vi "Single Axis Controller.vi"(0 "Measured Value":sgl, 1 "Setpoint\nSource":T3(radio), 2 "Signal\nParameters":T2, 3 "Manual\nSetpoint":sgl(slide) scale=-10.0..10.0, 4 "Enable":T1, 5 "Gains":cluster{"P":sgl, "I":sgl, "D":sgl}={"P"=0.1, "I"=0.1, "D"=0.1}, 9 "Integral In":sgl) -> (11 "Integral Out":sgl, 14 "Controller \nOutput":sgl, 15 "Sepoint \nChart":cluster{sgl, "Setpoint out":sgl}(graph), 16 "Output\nComponents\nChart":cluster{sgl, sgl, sgl, sgl, sgl, sgl}(graph), 19 "Waveform Chart":cluster{sgl, sgl}(graph))   [LabVIEW 2014]
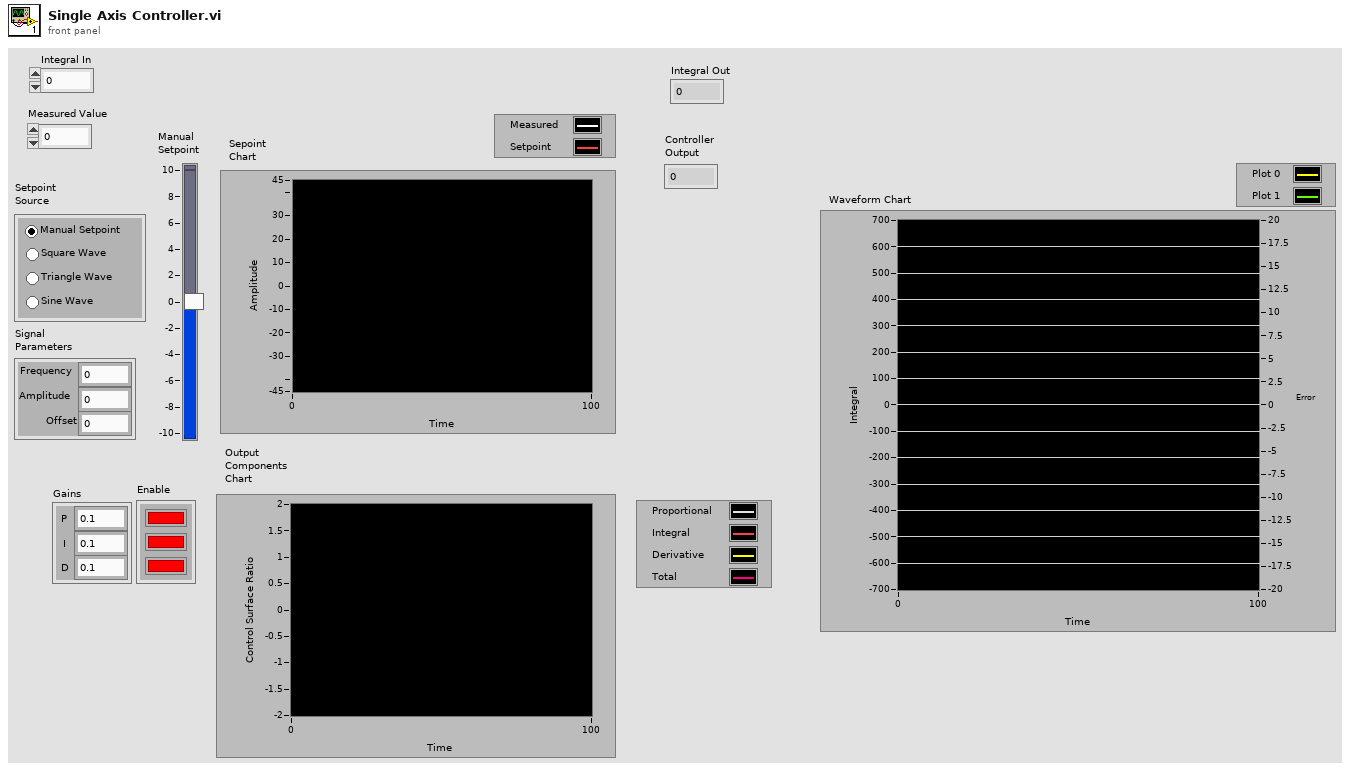
[diagram p1: front panel]
types:
  T1 = cluster{"P Enable":bool, "I Enable":bool, "D Enable":bool}
  T2 = cluster{"Frequency":sgl, "Amplitude":sgl, "Offset":sgl}
  T3 = enum32{"Manual Setpoint", "Square Wave", "Triangle Wave", "Sine Wave"}
  T4 = cluster{"Measured Value":sgl, "Setpoint out":sgl}
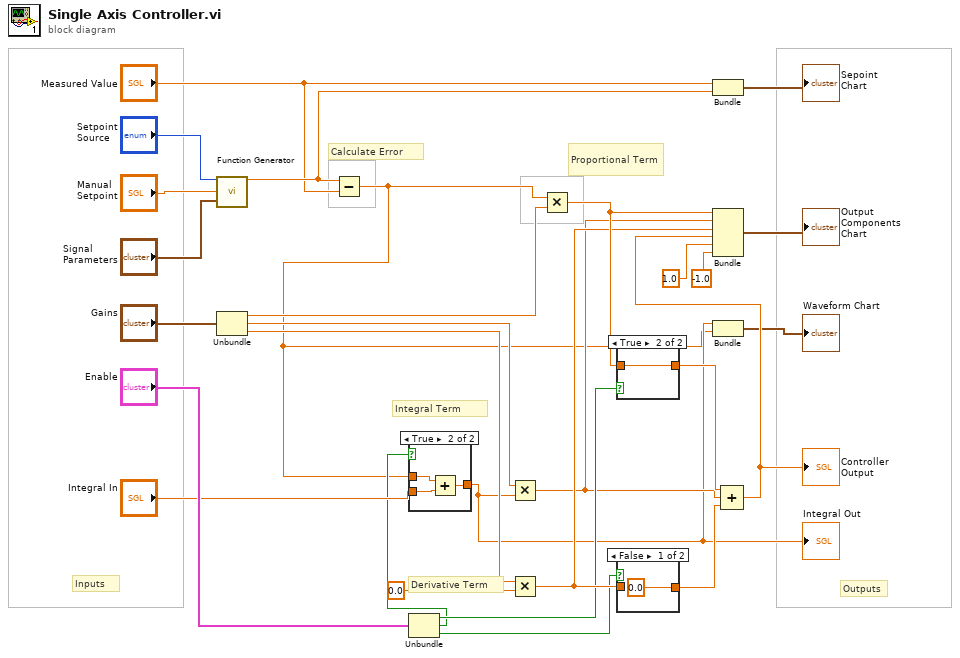
[diagram p0: block diagram]
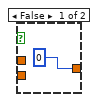
[diagram p3: hidden frame]
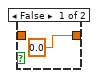
[diagram p4: hidden frame]
diagram:
  # "Proportional Term"
  # "Derivative Term"
  # "Integral Term"
  # "Calculate Error"
  # "Outputs"
  # "Inputs"
  n1 = call "Function Generator.vi"("Setpoint Source"="Setpoint\nSource", "Manual \nSetpoint in"="Manual\nSetpoint", "Signal\nParameters"="Signal\nParameters") -> ("Setpoint out"=w27:sgl)  [unwired: 12 in]
  n2 = Unbundle("Gains") -> ("P"=w21:sgl, "I"=w12:sgl, "D"=w11:sgl)
  n3 = Subtract(x=w27, y="Measured Value") -> (x-y=w1:sgl)
  n4 = Unbundle("Enable") -> ("P Enable"=w8:bool, "I Enable"=w2:bool, "D Enable"=w7:bool)
  n5 = case shown="True" w2 {
    tunnel: [0 w32] -> w4
    tunnel: w1 -> [_ w31]
    tunnel: "Integral In" -> [_ w30]
    frame False {
    }
    frame True {
      n6 = Add(x=w31, y=w30) -> (x+y=w32:sgl)
    }
  }
  "Integral Out" <- w4
  n7 = Multiply(x=w12, y=w4) -> (x*y=w6:sgl)
  n8 = Multiply(x=w11, y=sgl 0.0) -> (x*y=w13:sgl)
  n9 = Multiply(x=w1, y=w21) -> (x*y=w14:sgl)
  n10 = case shown="True" w8 {
    tunnel: w14 -> [_ w34]
    tunnel: [sgl 0.0 w34] -> w20
    frame False {
    }
    frame True {
    }
  }
  n11 = case shown="False" w7 {
    tunnel: [sgl 0.0 w36] -> w19
    tunnel: w13 -> [_ w36]
    frame False {
    }
    frame True {
    }
  }
  n12 = Bundle("Measured Value"="Measured Value", "Setpoint out"=w27) -> (→"Sepoint \nChart":T4)  [unwired: 1 in]
  n13 = Bundle(w4, w1) -> (→"Waveform Chart":cluster{sgl, sgl})  [unwired: 1 in]
  n14 = Compound Arithmetic op=ADD(w20, w6, w19) -> (w15:sgl)
  "Controller \nOutput" <- w15
  n15 = Bundle(w14, w6, w13, w15, sgl 1.0, sgl -1.0) -> (→"Output\nComponents\nChart":cluster{sgl, sgl, sgl, sgl, sgl, sgl})  [unwired: 1 in]
